vi "week_two.vi"() -> ()   [LabVIEW 2017]
panel:
  out "XY Graph":cluster{"Y":dbl[], "Y":dbl[]}[](graph)
  out "input":dbl(knob) scale=0.0..10.0
  out "output voltage":dbl(knob) scale=0.0..10.0
  in  "increment":dbl
  in  "maximum":dbl
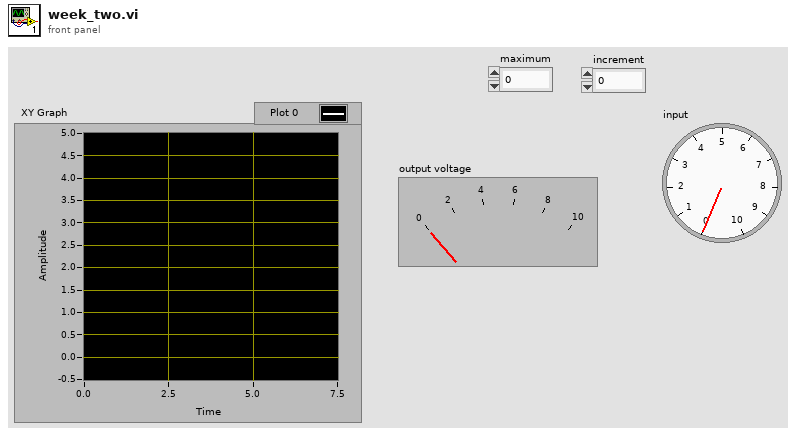
[diagram p1: front panel]
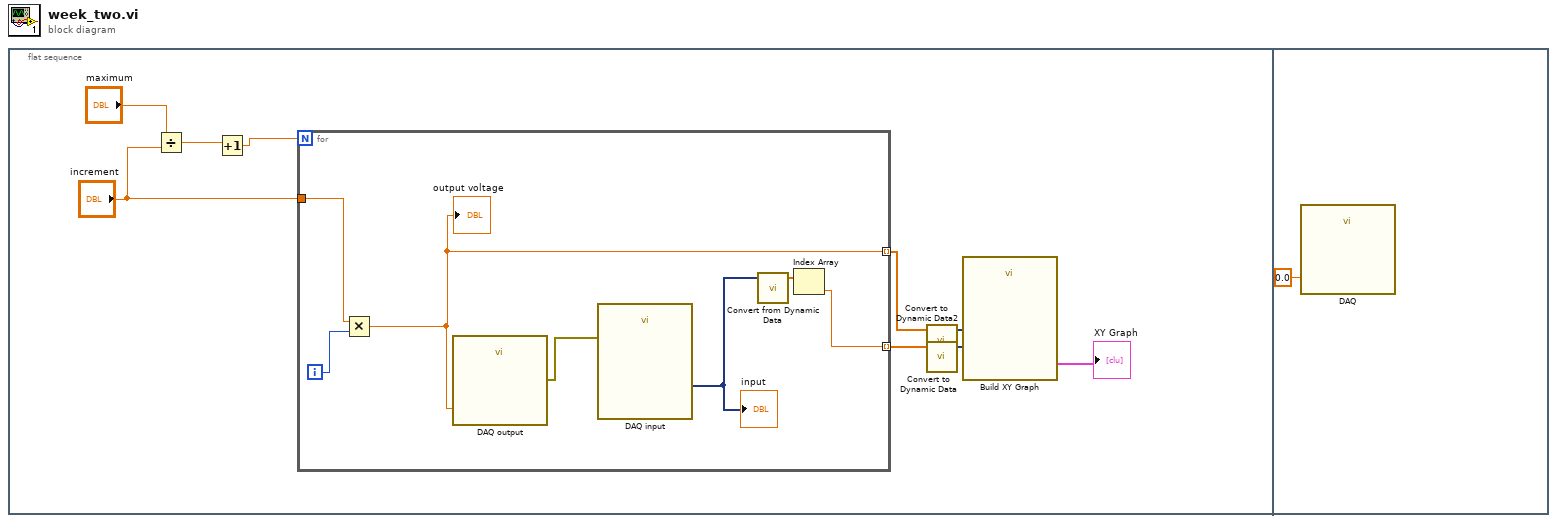
[diagram p0: block diagram]
diagram:
  n1 = flat-sequence {
    frame #0 {
      n2 = Divide(x="maximum", y="increment") -> (x/y=w2:dbl)
      n3 = Increment(x=w2) -> (x+1=w1:dbl)
      n4 = for {
        N: w1 -> [_]
        tunnel: "increment" -> [w15]
        tunnel: [w12] -> w6 mode=indexing
        tunnel: [w10] -> w4 mode=indexing
        i -> [w16]
        n5 = Multiply(x=w15, y=w16) -> (x*y=w10:dbl)
        "output voltage" <- w10
        n6 = call "DAQ output"("data"=w10) -> ("error out"=w11:errorcluster)  [unwired: 17 in, 1 out]
        n7 = call "DAQ input"("error in"=w11) -> ("data"=w14:dynamicdata)  [unwired: 16 in, 2 out]
        "input" <- w14
        n8 = call "Convert from Dynamic Data"("Dynamic Data Type"=w14) -> ("Array"=w13:dbl[])  [unwired: 3 in]
        n9 = Index Array(array=w13) -> (element=w12:dbl)  [unwired: 1 in]
      }
      n10 = call "Convert to Dynamic Data2"("Array"=w4) -> ("Dynamic Data Type"=w3:dynamicdata)  [unwired: 3 in]
      n11 = call "Convert to Dynamic Data"("Array"=w6) -> ("Dynamic Data Type"=w5:dynamicdata)  [unwired: 3 in]
      n12 = call "Build XY Graph"("Y Input"=w5, "X Input"=w3) -> ("XY Graph"=→"XY Graph":cluster{"X":dbl[], "Y":dbl[]}[])  [unwired: 8 in, 1 out]
    }
    frame #1 {
      n13 = call "DAQ"("data"=0.0) -> ()  [unwired: 17 in, 2 out]
    }
  }
